vi "Read Active Funnel.vi"(8 "error in (no error)":errorcluster, 11 "Setting Database in":refnum<class "Setting Database.lvclass">) -> (0 "error out":errorcluster, 2 "Active Funnel":refnum<class "Funnel Settings.lvclass">, 3 "Setting Database out":refnum<class "Setting Database.lvclass">)   [LabVIEW 2019, in "Setting Database.lvclass"]
uses:
  Setting Database.lvclass
  Funnel Settings/Funnel Settings.lvclass
  C:/Users/Albro/Documents/GitHub/AFM-Lithography/lvsrc/Classes/Settings/ObjectSettings/ObjectSettings.lvclass
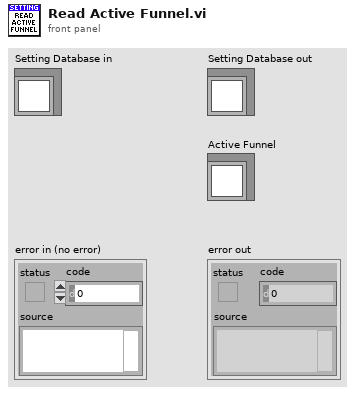
[diagram p1: front panel]
types:
  T1 = cluster{"Path":string, "Funnel":string, "Rectangle":string, "Dot":string}
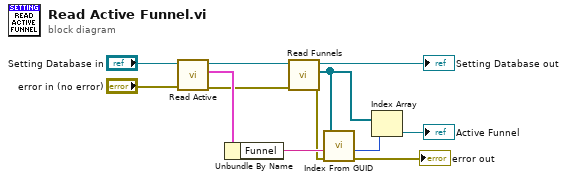
[diagram p0: block diagram]
diagram:
  n1 = call "Read Active.vi"("error in (no error)"="error in (no error)", "Setting Database in"="Setting Database in") -> ("error out"=w6:errorcluster, "Active"=w8:T1, "Setting Database out"=w9:refnum<class "Setting Database.lvclass">)  [unwired: 7 in]
  n2 = Unbundle By Name(w8) -> ("Funnel"=w4:string)
  n3 = call "Read Funnels.vi"("error in (no error)"=w6, "Setting Database in"=w9) -> ("error out"=w2:errorcluster, "Funnels"=w5:refnum<class "Funnel Settings.lvclass">[], "Setting Database out"=→"Setting Database out":refnum<class "Setting Database.lvclass">)  [unwired: 7 in]
  n4 = call "Index From GUID.vi"("error in"=w2, "GUID"=w4, "Objects In"=w5) -> ("error out"=→"error out":errorcluster, "Index"=w3:i32)  [unwired: 5 in, 2 out]
  n5 = Index Array(array=w5, index=w3) -> (element=→"Active Funnel":refnum<class "Funnel Settings.lvclass">)
